vi "load_kbolott_volume.vi"(1 "HBCmPath":string="C:\\LABVIEW\\BLV DAC Range & Voltage\\LABVIEW\\BLV\\bolo_files\\standard_camHBCm_kbolott_and_volum_PV_new_.dat", 3 "SavePath":string="C:\\LABVIEW\\BLV DAC Range & Voltage\\LABVIEW\\BLV\\bolo_files\\kbolott_and_volum_PV_new.dat", 4 "VBClPath":string="C:\\LABVIEW\\BLV DAC Range & Voltage\\LABVIEW\\BLV\\bolo_files\\standard_camVBCl_kbolott_and_volum_PV_new_.dat", 5 "VBCrPath":string="C:\\LABVIEW\\BLV DAC Range & Voltage\\LABVIEW\\BLV\\bolo_files\\standard_camVBCr_kbolott_and_volum_PV_new_.dat") -> (2 "output":dbl[][](array[numeric])=[[1e-05, 1e-05], [9.8364458e-05, 1.8160732], [0.00029863964, 770.25441], [0.00053910452, 1653.5432], [0.00071569496, 2554.7619], [0.00083348142, 3356.1809], [0.00092645429, 4021.9678], [0.00099241932, 4570.4466], [0.0010332482, 4989.6792], [0.0010552469, 5170.4882], [0.0010669981, 5192.5645], [0.001071534, 5152.6222], [0.0010766644, 5109.6704], [0.0010841289, 5094.9972], [0.0010884845, 5078.237], [0.0010888843, 5058.9416], [0.0010882289, 5056.581], [0.0010872861, 5078.1684], [0.0010832221, 5096.5196], [0.0010760805, 5113.7904], [0.0010685167, 5141.4566], [0.0010644166, 5189.7831], [0.0010539441, 5182.7365], [0.0010337779, 5034.6928], [0.00098716411, 4625.8518], [0.00091599422, 4090.3707], [0.00082376071, 3438.9665], [0.00070194108, 2659.5109], [0.00051785958, 1753.3355], [0.00030745544, 937.82125], [0.00014081292, 59.55205], [1e-05, 1e-05], [0.0, 0.0], [0.0, 0.0], [0.0, 0.0], [0.0, 0.0], [0.0, 0.0], [0.0, 0.0], [0.0, 0.0], [0.0, 0.0], [0.0, 0.0], [0.0, 0.0], [0.0, 0.0], [0.0, 0.0], [0.0, 0.0], [0.0, 0.0], [0.0, 0.0], [0.0, 0.0], [0.0019134875, 3474.3085], [0.0020594744, 3690.1455], [0.002175929, 3861.3028], [0.0022530617, 3956.5918], [0.0023492529, 4057.9903], [0.0024581424, 4205.0841], [0.0025383764, 4324.9746], [0.0025876415, 4417.9525], [0.0026676725, 4566.0612], [0.0027635964, 4770.6296], [0.0028188521, 4914.295], [0.0028263806, 4970.0105], [0.0028491244, 5014.7926], [0.0028762033, 5060.279], [0.0028430703, 4969.1072], [0.0027058578, 4592.2853], [0.0019047772, 4936.5706], [0.0023594746, 6388.5028], [0.0025094117, 6336.5413], [0.002569351, 6048.9284], [0.0026367277, 5794.3031], [0.002714522, 5668.1597], [0.0027530637, 5505.217], [0.0027520905, 5312.6378], [0.0027781484, 5183.8321], [0.0028283925, 5165.5044], [0.0028425709, 5118.655], [0.00281436, 5016.5122], [0.0027996491, 4909.784], [0.0027993913, 4845.125], [0.0027603692, 4728.4661], [0.0026886073, 4585.7454], [0.0026437627, 4495.4419], [0.0026242501, 4486.7206], [0.0025685332, 4434.986], [0.0024747416, 4324.8822], [0.0023915919, 4209.8149], [0.002319616, 4111.844], [0.0022042921, 3923.4955], [0.0020485146, 3644.5259], [0.0024033884, 3597.1969], [0.002066694, 2566.1598], [0.0017718795, 1878.4004], [0.0015136288, 1414.3006], [0.0013043692, 1094.5581], [0.0011378765, 882.65731], [0.00097324167, 712.97006], [0.00080739571, 571.52867], [0.0, 0.0], [0.0, 0.0], [0.0, 0.0], [0.0, 0.0], [0.0, 0.0], [0.0, 0.0], [0.0, 0.0], [0.0, 0.0], [0.0, 0.0], [0.0, 0.0], [0.0, 0.0], [0.0, 0.0], [0.0, 0.0], [0.0, 0.0], [0.0, 0.0], [0.0, 0.0], [0.0, 0.0], [0.0, 0.0], [0.0, 0.0], [0.0, 0.0], [0.0, 0.0], [0.0, 0.0], [0.0, 0.0], [0.0, 0.0], [0.0, 0.0], [0.0, 0.0], [0.0, 0.0], [0.0, 0.0], [0.0, 0.0], [0.0, 0.0], [0.0, 0.0], [0.0, 0.0]])   [LabVIEW 2014]
uses:
  <vilib>/Analysis/Matrix/Datatypes/RealMatrix.ctl
  <vilib>/Utility/file.llb/Read From Spreadsheet File (DBL).vi
  <vilib>/Utility/file.llb/Write To Spreadsheet File (DBL).vi
  <vilib>/Analysis/Matrix/NI_Matrix.lvlib
panel:
  in  "DEBUG AT 1-4":string="6"
  out "TMP":T1
  in  "DEBUG":bool=TRUE
  out "VBCr Import":T1
  out "VBCl Import (0-16)":T1
  out "VBCl Import (17-24)":T1
  out "HBCm Import":T1
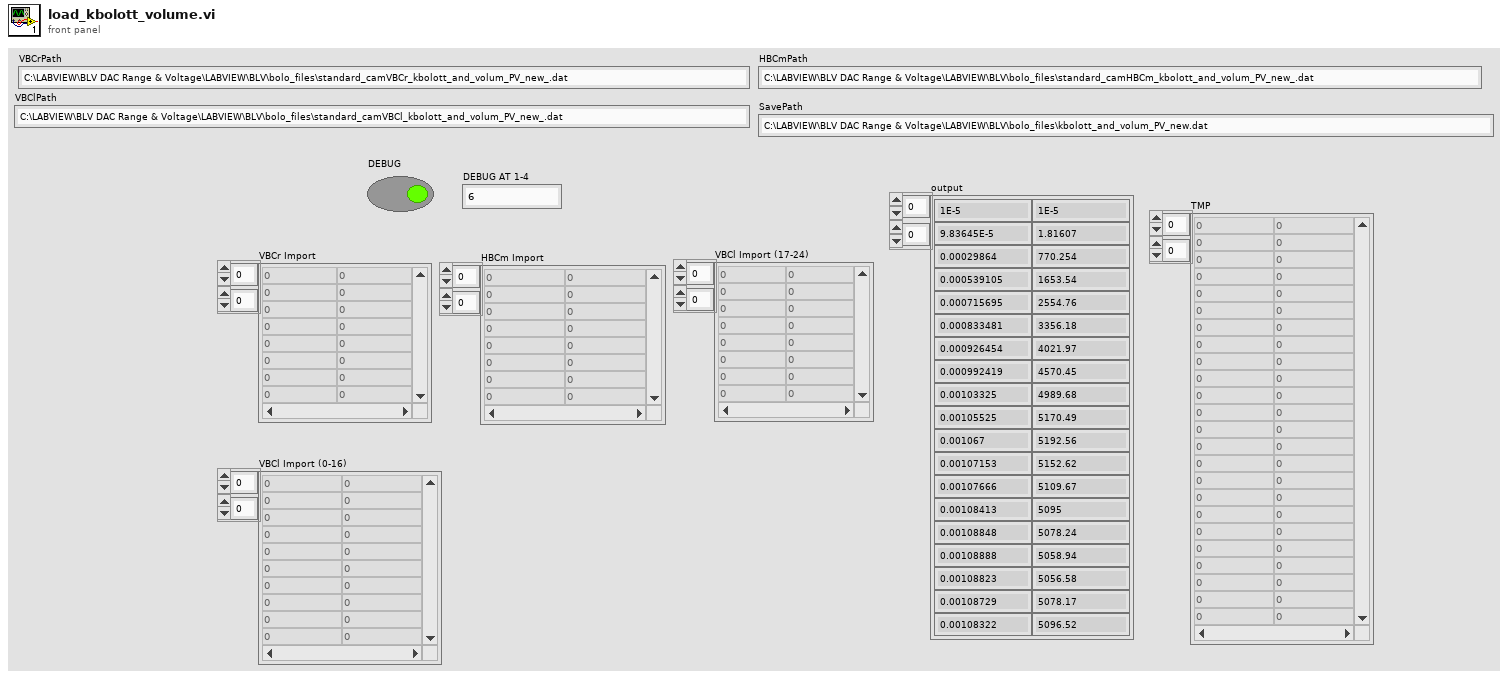
[diagram p1: front panel]
types:
  T1 = typedef "NI_Matrix.lvlib/RealMatrix.ctl" = dbl[][]
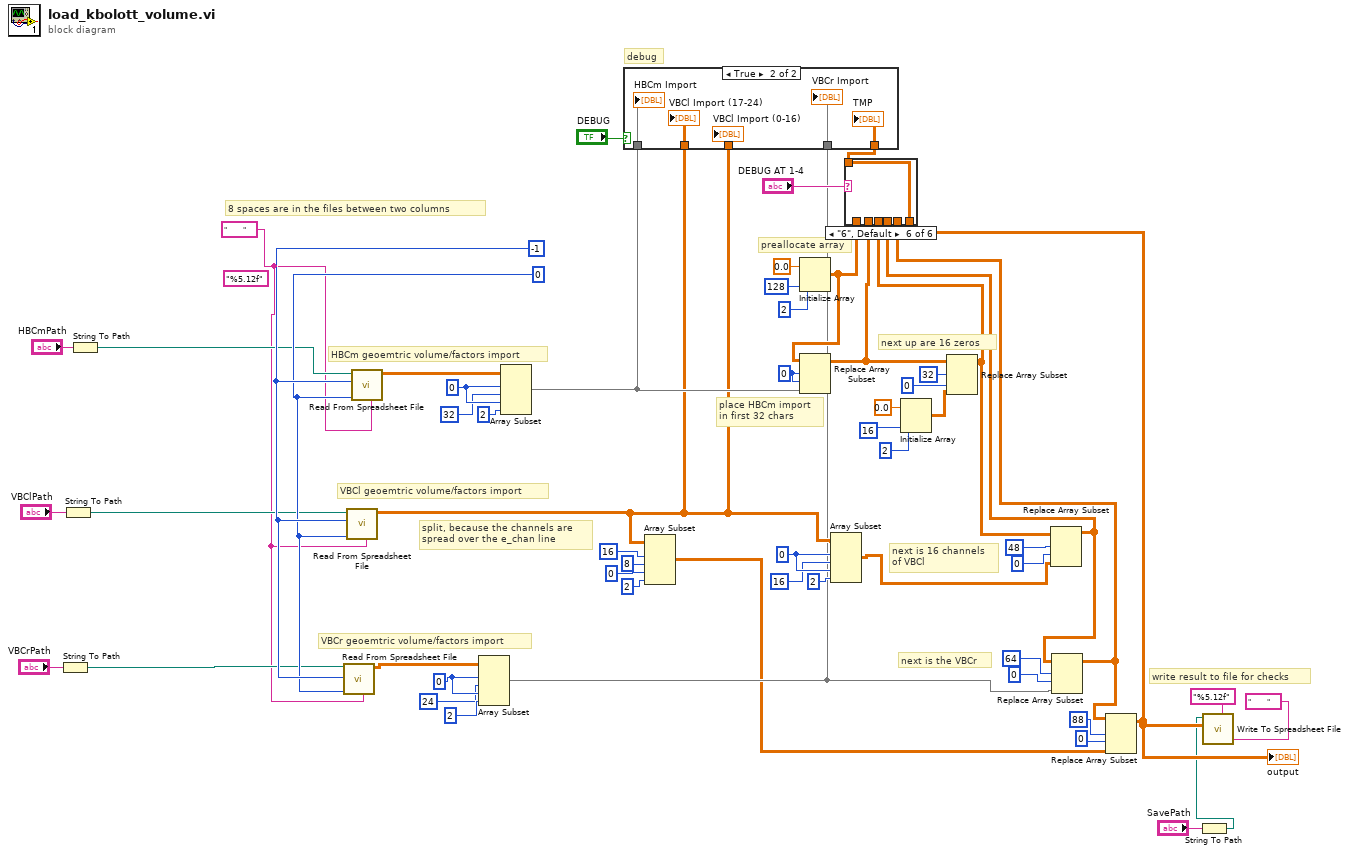
[diagram p0: block diagram]
diagram:
  w38 = 0 ("index (row)")
  w44 = 0
  w51 = 0
  w58 = 0
  w1 = "        "
  w47 = 0
  (unwired) "%5.12f"
  w48 = -1
  # "write result to file for checks"
  # "next is the VBCr"
  # "next is 16 channels\nof VBCl"
  # "next up are 16 zeros"
  # "place HBCm import\nin first 32 chars"
  # "preallocate array"
  # "split, because the channels are\nspread over the e_chan line"
  # "VBCr geoemtric volume/factors import"
  # "VBCl geoemtric volume/factors import"
  # "HBCm geoemtric volume/factors import"
  # "debug"
  # "8 spaces are in the files between two columns"
  n1 = String To Path(string="VBCrPath") -> (path=w2:path)
  n2 = String To Path(string="VBClPath") -> (path=w7:path)
  n3 = String To Path(string="HBCmPath") -> (path=w6:path)
  n4 = call-poly <vilib>:"Read From Spreadsheet File.vi"("delimiter (\\t)"=w1, "max characters/row  (no limit:0)"=w47, "number of rows (all:-1)"=w48, "file path (dialog if empty)"=w2) -> ("all rows"=w45:dbl[][])  [unwired: 3 in, 4 out]
  n5 = call-poly <vilib>:"Read From Spreadsheet File.vi"("delimiter (\\t)"=w1, "max characters/row  (no limit:0)"=w47, "number of rows (all:-1)"=w48, "file path (dialog if empty)"=w7) -> ("all rows"=w29:dbl[][])  [unwired: 3 in, 4 out]
  n6 = call-poly <vilib>:"Read From Spreadsheet File.vi"("delimiter (\\t)"=w1, "max characters/row  (no limit:0)"=w47, "number of rows (all:-1)"=w48, "file path (dialog if empty)"=w6) -> ("all rows"=w46:dbl[][])  [unwired: 3 in, 4 out]
  n7 = Array Subset(array=w45, index (row)=w44, length (row)=24, index (col)=w44, length (col)=2) -> (w21:dbl[][])
  n8 = Array Subset(array=w46, index (row)=w51, length (row)=32, index (col)=w51, length (col)=2) -> (w30:dbl[][])
  n9 = Array Subset(array=w29, index (row)=16, length (row)=8, index (col)=0, length (col)=2) -> (w15:dbl[][])
  n10 = Initialize Array(0.0 ("element"), 128 ("dimension size"), 2 ("dimension size")) -> (w26:dbl[][])
  n11 = Replace Array Subset(array=w26, new element=w30, index (row)=w38, index (col)=w38) -> (w24:dbl[][])
  n12 = Array Subset(array=w29, index (row)=w58, length (row)=16, index (col)=w58, length (col)=2) -> (w22:dbl[][])
  n13 = Initialize Array(0.0 ("element"), 16 ("dimension size"), 2 ("dimension size")) -> (w27:dbl[][])
  n14 = Replace Array Subset(array=w24, new element=w27, index (row)=32, index (col)=0 ("disabled index (col)")) -> (w18:dbl[][])
  n15 = Replace Array Subset(array=w18, new element=w22, index (row)=48, index (col)=0 ("disabled index (col)")) -> (w17:dbl[][])
  n16 = Replace Array Subset(array=w17, new element=w21, index (row)=64, index (col)=0 ("disabled index (col)")) -> (w16:dbl[][])
  n17 = Replace Array Subset(array=w16, new element=w15, index (row)=88, index (col)=0 ("disabled index (col)")) -> (w11:dbl[][])
  "output" <- w11
  n18 = case shown="\"6\", Default" "DEBUG AT 1-4" {
    tunnel: w26 -> [w59 _ _ _ _ _]
    tunnel: [w59 w60 w61 w62 w63 w64] -> w25
    tunnel: w24 -> [_ w60 _ _ _ _]
    tunnel: w18 -> [_ _ w61 _ _ _]
    tunnel: w17 -> [_ _ _ w62 _ _]
    tunnel: w16 -> [_ _ _ _ w63 _]
    tunnel: w11 -> [_ _ _ _ _ w64]
    frame "1" {
    }
    frame "2" {
    }
    frame "3" {
    }
    frame "4" {
    }
    frame "5" {
    }
    frame "6", Default {
    }
  }
  n19 = case shown="True" "DEBUG" {
    tunnel: w30 -> [_ w69]
    tunnel: w29 -> [_ w68]
    tunnel: w29 -> [_ w67]
    tunnel: w21 -> [_ w66]
    tunnel: w25 -> [_ w65]
    frame False {
    }
    frame True {
      "VBCr Import" <- w66
      "HBCm Import" <- w69
      "VBCl Import (17-24)" <- w68
      "VBCl Import (0-16)" <- w67
      "TMP" <- w65
    }
  }
  n20 = String To Path(string="SavePath") -> (path=w5:path)
  n21 = call-poly <vilib>:"Write To Spreadsheet File.vi"("delimiter (\\t)"="        " ("delimiter (\\t)"), "format (%.3f)"="%5.12f", "2D data"=w11, "file path (dialog if empty)"=w5) -> ()  [unwired: 4 in, 1 out]
